vi "D2SParser - Private - Function - Read Character Name.vi"(8 "error in (no error)":errorcluster, 11 "D2SParser in":refnum<class "D2SParser.lvclass">) -> (0 "error out":errorcluster, 3 "D2SParser out":refnum<class "D2SParser.lvclass">)   [LabVIEW 2015, in "D2SParser.lvclass"]
uses:
  D2SParser.lvclass
  D2SParser.lvclass/D2SParser.ctl
  D2Character/D2Character.lvclass/D2Character.ctl
  D2Character/D2Character - Accessors - Set Name.vi
  D2SParser - Private - Helper - Read ASCII.vi
  D2Character/D2Character.lvclass
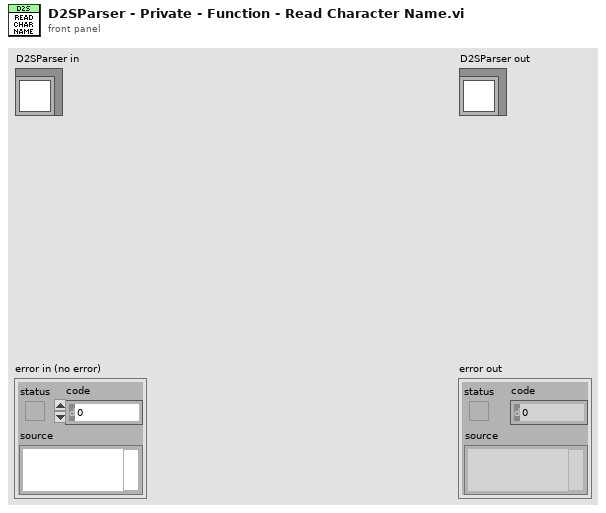
[diagram p1: front panel]
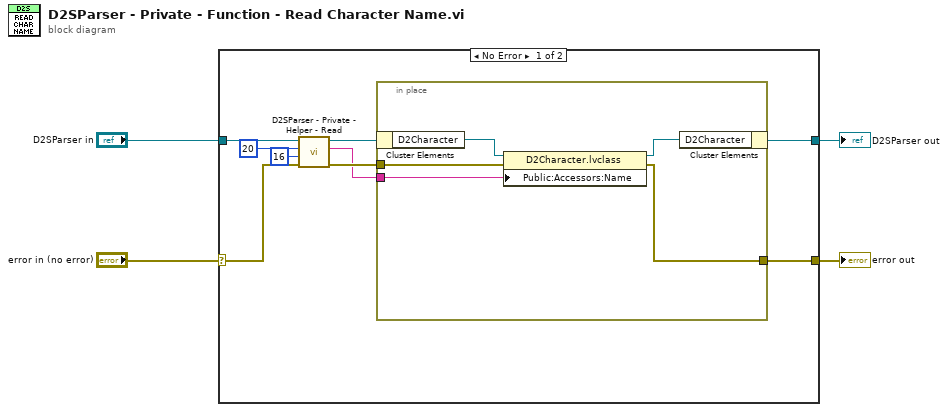
[diagram p0: block diagram]
diagram:
  n1 = case shown="No Error" "error in (no error)" {
    selector: "error in (no error)" -> [w12 w20]
    tunnel: [w9 w20] -> w3
    tunnel: [w8 w19] -> w1
    tunnel: "D2SParser in" -> [w13 w19]
    frame No Error {
      n2 = call-poly "D2SParser - Private - Helper - Read.vi"("error in (no error)"=w12, "# Characters"=16, "Position"=i64 20, "D2SParser in"=w13) -> ("error out"=w10:errorcluster, "ASCII"=w5:string, "D2SParser out"=w11:refnum<class "D2SParser.lvclass">)  [unwired: 5 in]
      n3 = in-place {
        in-place-border: w10 -> [w16]
        in-place-border: [w15] -> w9
        in-place-border: w5 -> [w14]
        n4 = in-place-cluster #1(w11) -> ("D2Character"=w18:refnum<class "D2Character.lvclass">)
        n5 = property class="D2Character.lvclass"(reference=w18, error in=w16, "Public:Accessors:Name"=w14) -> (reference out=w17:refnum<class "D2Character.lvclass">, error out=w15:errorcluster)
        n6 = in-place-cluster #1("D2Character"=w17) -> (w8:refnum<class "D2SParser.lvclass">)
      }
    }
    frame Error {
    }
  }
  "error out" <- w3
  "D2SParser out" <- w1
